vi "Rename AO Endpoint.vi"(8 "error in (no error)":errorcluster, 9 "New name":string, 10 "Old name":string, 11 "Tosca in":refnum<class "Parameters.lvclass">) -> (0 "error out":errorcluster, 3 "Tosca out":refnum<class "Parameters.lvclass">)   [LabVIEW 2020, in "Parameters.lvclass"]
uses:
  Parameters.lvclass
  Parameters.lvclass/Parameters.ctl
  State/State.lvclass/State.ctl
  State/Read SigMan.vi
  State/Write SigMan.vi
  epl-vi-lib/Signal Synthesis VIs/4th Generation/Classes/SignalManager/SignalManager.lvclass
  State/State.lvclass
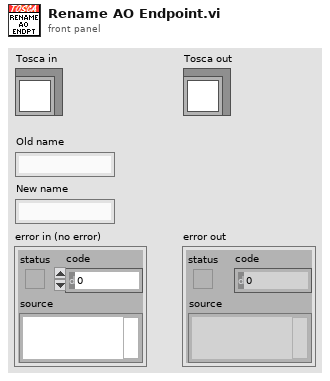
[diagram p1: front panel]
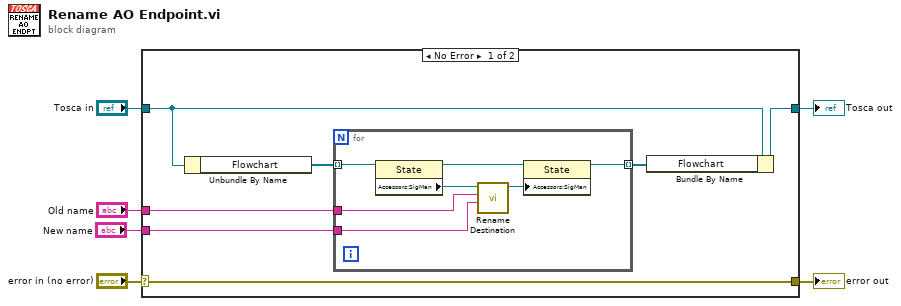
[diagram p0: block diagram]
diagram:
  n1 = case shown="No Error" "error in (no error)" {
    selector: "error in (no error)" -> [w13 w22]
    tunnel: [w13 w22] -> w5
    tunnel: [w10 w21] -> w3
    tunnel: "Tosca in" -> [w12 w21]
    tunnel: "Old name" -> [w8 _]
    tunnel: "New name" -> [w7 _]
    frame No Error {
      n2 = Unbundle By Name(w12) -> ("Flowchart"=w11:refnum<class "State.lvclass">[])
      n3 = for {
        tunnel: w11 -> [w20] mode=indexing
        tunnel: [w16] -> w9 mode=indexing
        tunnel: w8 -> [w15]
        tunnel: w7 -> [w14]
        n4 = property class="State"(reference=w20) -> (reference out=w18:refnum<class "State.lvclass">, "Accessors:SigMan"=w19:refnum<class "SignalManager.lvclass">)  [unwired: 1 in, 1 out]
        n5 = call "Rename Destination.vi"("New name"=w14, "Old name"=w15, "SigMan in"=w19) -> ("SigMan out"=w17:refnum<class "SignalManager.lvclass">)  [unwired: 7 in, 1 out]
        n6 = property class="State"(reference=w18, "Accessors:SigMan"=w17) -> (reference out=w16:refnum<class "State.lvclass">)  [unwired: 1 in, 1 out]
      }
      n7 = Bundle By Name(cluster=w12, "Flowchart"=w9) -> (w10:refnum<class "Parameters.lvclass">)
    }
    frame Error {
    }
  }
  "error out" <- w5
  "Tosca out" <- w3
